vi "Init.vi"(8 "error in (no error)":errorcluster) -> (0 "error out":errorcluster)   [LabVIEW 2026, in "TALOS.lvlib" / "Classes.lvlib" / "Error Filter.lvclass"]
uses:
  Error Filter.lvclass
  Support VIs/Global Memory.vi
  TALOS.lvlib
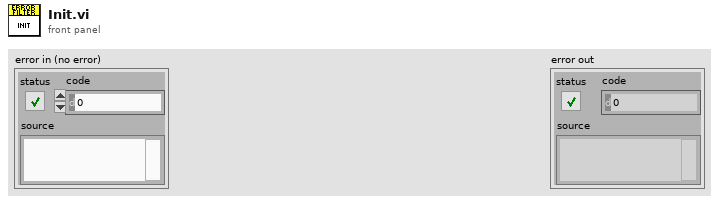
[diagram p1: front panel]
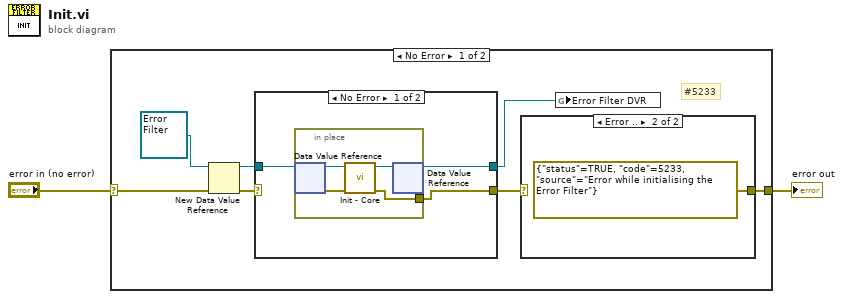
[diagram p0: block diagram]
diagram:
  n1 = case shown="No Error" "error in (no error)" {
    selector: "error in (no error)" -> [w6 w21]
    tunnel: [w3 w21] -> w1
    frame No Error {
      # "#5233"
      n2 = New Data Value Reference(data value=refnum<class "Error Filter.lvclass"> refnum ("Error Filter in"), error in=w6) -> (data value reference=w8:refnum<data-value>, error out=w7:errorcluster)
      n3 = case shown="No Error" w7 {
        selector: w7 -> [_ w20]
        tunnel: w8 -> [w14 w19]
        tunnel: [w12 w20] -> w4
        tunnel: [w13 w19] -> w5
        frame No Error {
          n4 = in-place {
            in-place-border: [w16] -> w12
            n5 = in-place-dvr #1(w14) -> (w18:refnum<class "Error Filter.lvclass">, w15:errorcluster)
            n6 = call "Init - Core.vi"("error in (no error)"=w15, "Error Filter in"=w18) -> ("error out"=w16:errorcluster, "Error Filter out"=w17:refnum<class "Error Filter.lvclass">)  [unwired: 8 in]
            n7 = in-place-dvr #1(w17) -> (w13:refnum<data-value>)  [unwired: 1 out]
          }
        }
        frame Error {
        }
      }
      n8 = case shown="Error .." w4 {
        selector: w4 -> [w10 _]
        tunnel: [w10 errorcluster {"status"=TRUE, "code"=5233, "source"="Error while initialising the Error Filter"} ("error IO")] -> w3
        frame No Error {
        }
        frame Error {
        }
      }
      n9 = global write "Global Memory.vi" "Error Filter DVR"(w5) -> ()
    }
    frame Error {
    }
  }
  "error out" <- w1
